vi "Save_Ensight_Case.vi"() -> (5 "Plug in titles":string[](array[string]), 7 "Plug in values":string[](array[string]))   [LabVIEW 2011]
uses:
  Globals/Meas_global.vi
  <vilib>/Analysis/NI_AALBase.lvlib
panel:
  out "Channel Varaibles":string[](array[string])
  out "Variable Names":string[](array[string])
  out "File Paths":path[](array[path])
  out "Results Folder Exists?":bool
  # "You must have just these two indicators on the connector pane of the vi"
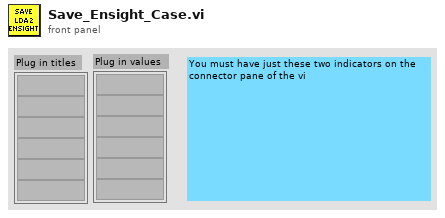
[diagram p1: front panel]
types:
  T1 = typedef "Analysis_info_cluster.ctl" = cluster{"Colour":u32, "Inst type":T2, "Inst name":string, "Symbol":string, "Code name":string, "Extra Info":string, "Inst Array":T3, "Index":i32, "Voltage Index":i32, "Extra Titles":string[], "Extra Values":string[], "Eng Values":dbl[], "Time (ms)":dbl[], "Voltage":dbl[], "U":dbl, "u^2":dbl, "u^3":dbl, "u^4":dbl, "Skew_u":dbl, "Kurt_u":dbl, "Sd Error in Mean":dbl, "% u'/U":dbl, "X":dbl, "Y":dbl, "Z":dbl, "Spectra":T4, "Autocorrelation":T4, "Timescale integral to 25%":dbl, "Sd Error in Variance":dbl, "Calib File":path, "Calib Constants":dbl[], "Histogram":T4, "Output Position":bool, "Full Stats":bool, "Weighting":dbl[]}
  T2 = typedef "Inst_type.ctl" = enum16{"Propeller anemometer", "Raw voltage", "Pressure Transducer", "Pitot-static tube", "Preston tube", "Hot wire", "Cross wire 1", "Cross wire 2", "Generic Linear", "Generic Polynomial", "Generic BackPoly", "Fast FID", "Thermocouple", "Cold wire", "Pulsed Wire", "LDA Vel", "LDA Tran time", "LDA Arr time"}
  T3 = typedef "Instrument_Array.ctl" = enum16{"PWA", "LDA", "Analogue"}
  T4 = typedef "XY_Plot_Cluster.ctl" = cluster{"First Name":string, "Second Name":string, "X axis name":string, "Y axis name":string, "X array":dbl[], "Y array":dbl[]}
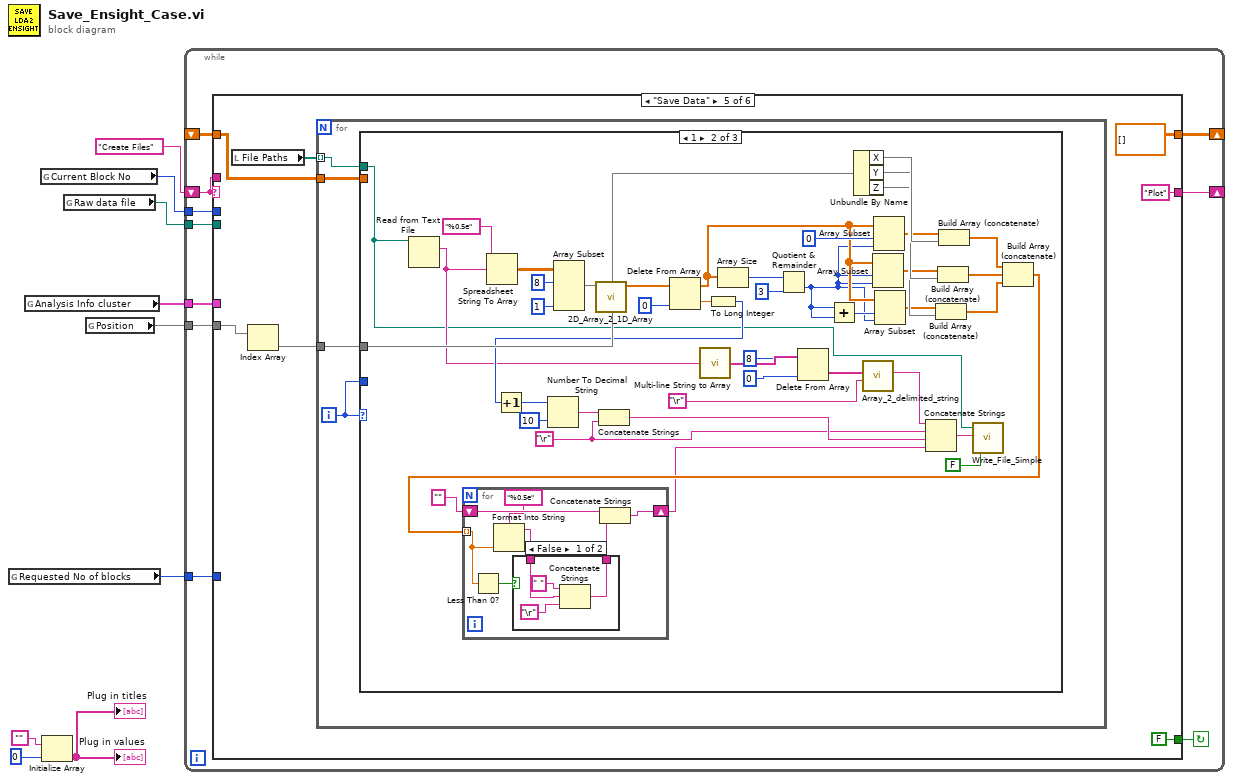
[diagram p0: block diagram]
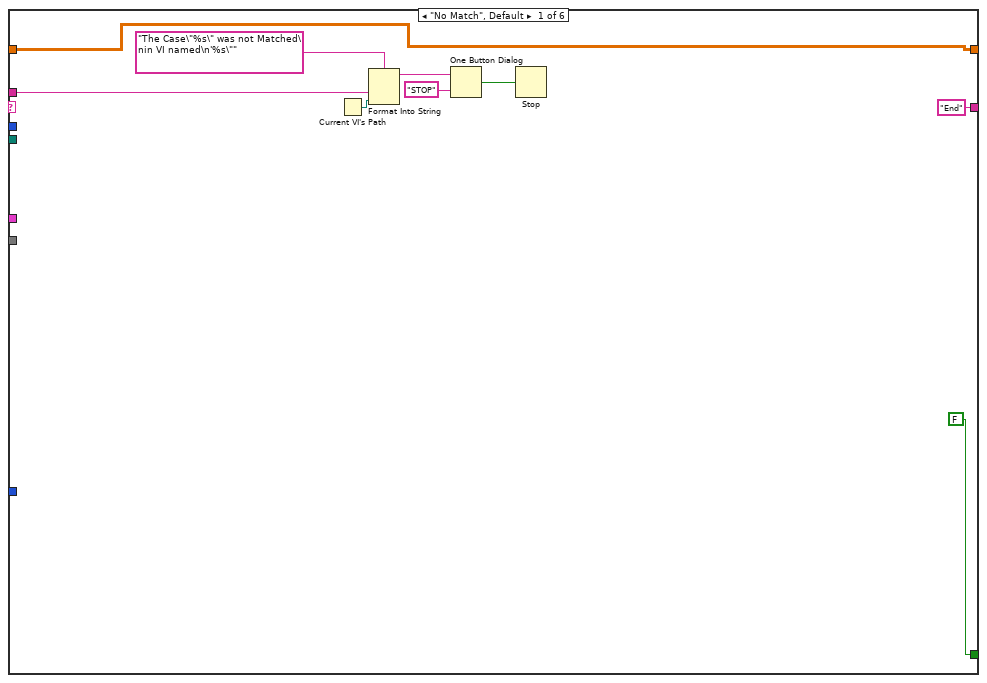
[diagram p2: hidden frame]
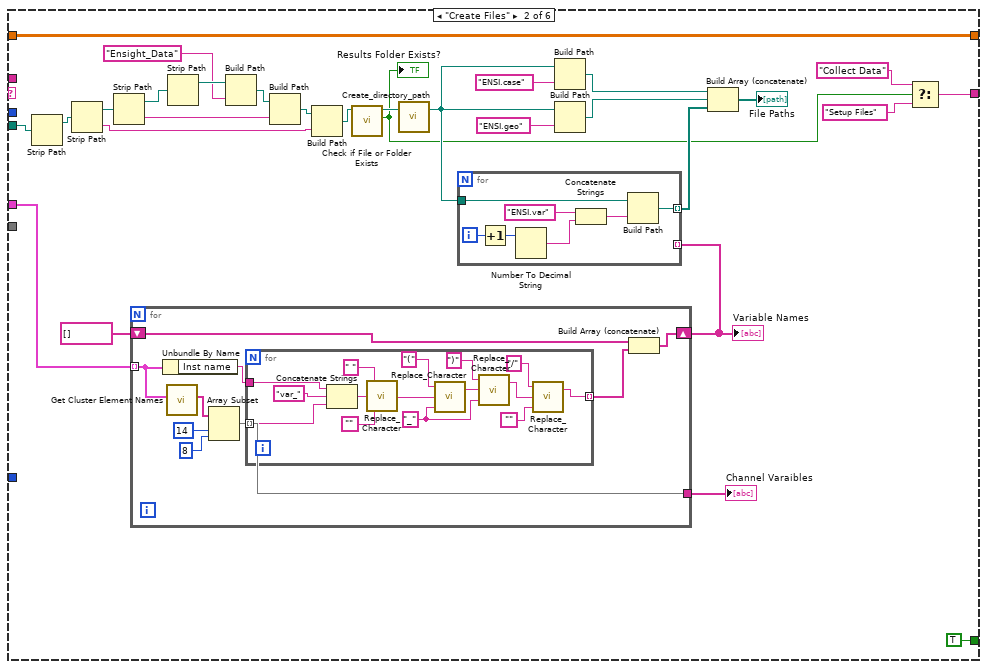
[diagram p3: hidden frame]
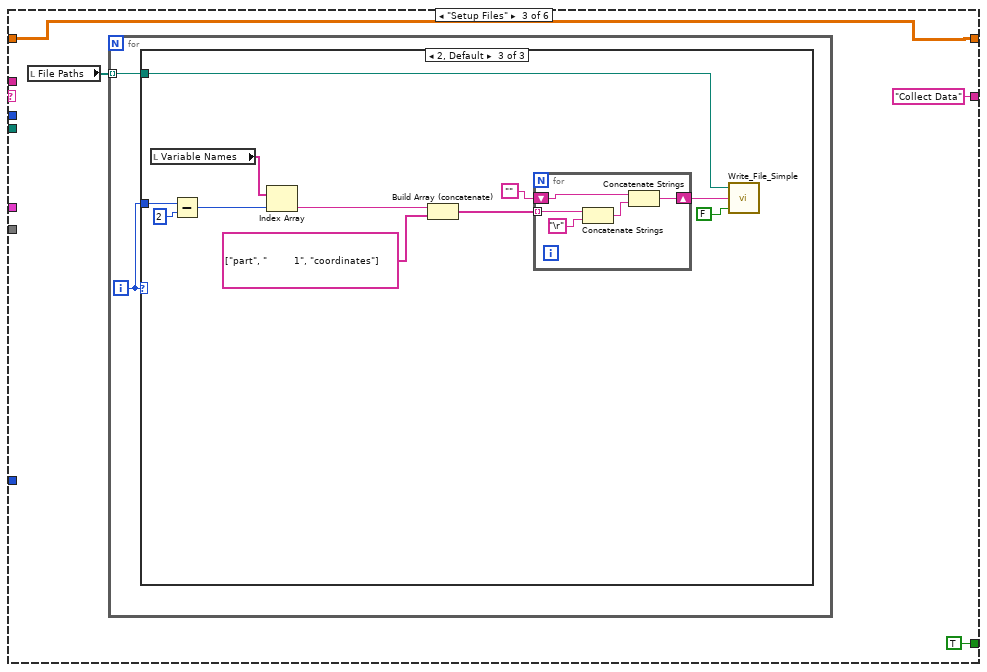
[diagram p4: hidden frame]
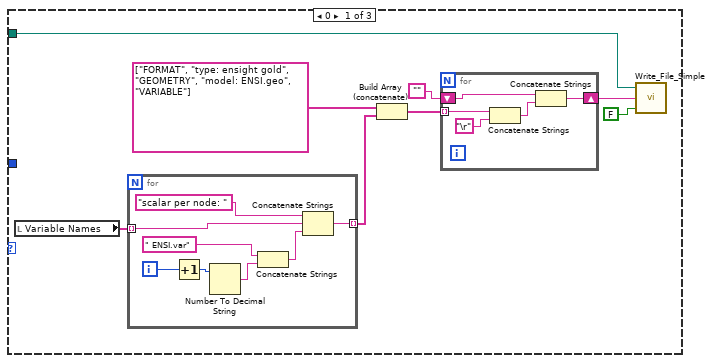
[diagram p5: hidden frame]
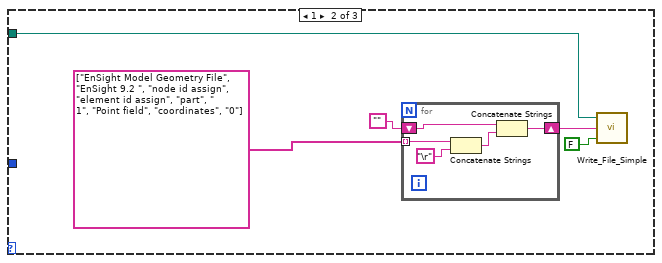
[diagram p6: hidden frame]
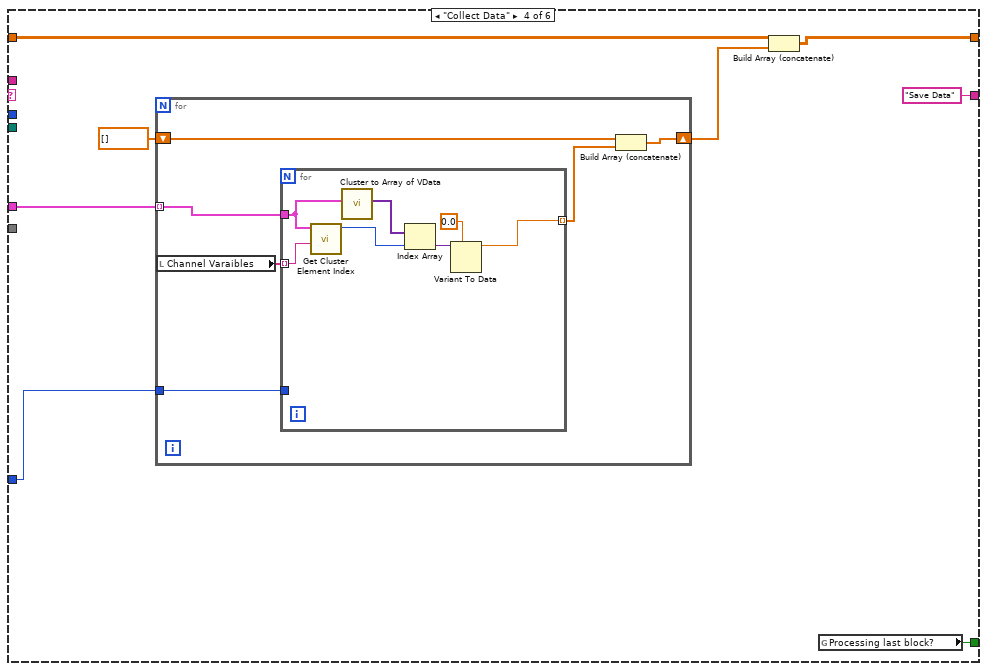
[diagram p7: hidden frame]
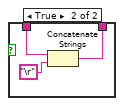
[diagram p9: hidden frame]
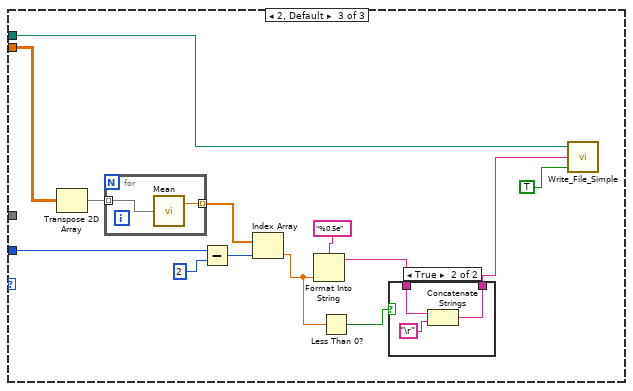
[diagram p10: hidden frame]
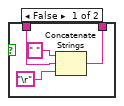
[diagram p11: hidden frame]
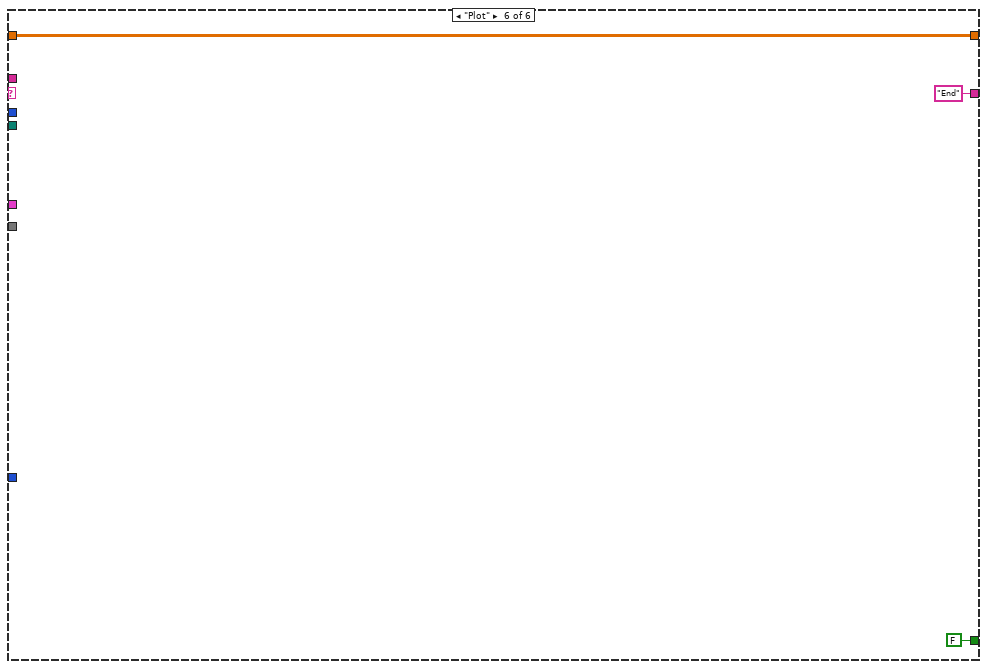
[diagram p12: hidden frame]
diagram:
  n1 = global read "Meas_global.vi" "Requested No of blocks"() -> (w2:i32)
  n2 = global read "Meas_global.vi" "Analysis Info cluster"() -> (w3:T1[])
  n3 = global read "Meas_global.vi" "Current Block No"() -> (w5:i32)
  n4 = Initialize Array("", 0) -> (→"Plug in values" →"Plug in titles":string[])
  n5 = global read "Meas_global.vi" "Raw data file"() -> (w4:path)
  n6 = global read "Meas_global.vi" "Position"() -> (w1)
  n7 = while {
    shift-left: "Create Files" -> [w19]
    shift-right: [w18] -> _
    tunnel: w5 -> [w16]
    tunnel: w4 -> [w15]
    tunnel: w3 -> [w14]
    tunnel: w2 -> [w13]
    tunnel: w1 -> [w12]
    shift-right: [w11] -> _
    shift-left: _ -> [w10]
    stop <- w17 continue-if-true
    n8 = case shown="\"Save Data\"" w19 {
      tunnel: ["End" ("t") w40 "Collect Data" ("t") "Save Data" ("t") "Plot" ("t") "End" ("t")] -> w18
      tunnel: w19 -> [w24 _ _ _ _ _]
      tunnel: [FALSE TRUE ("Processing last block?") TRUE ("Processing last block?") w149 FALSE ("Processing last block?") FALSE ("Processing last block?")] -> w17
      tunnel: w16 -> [_ _ _ _ _ _]
      tunnel: w15 -> [_ w57 _ _ _ _]
      tunnel: w14 -> [_ w36 _ w148 _ _]
      tunnel: w13 -> [_ _ _ w147 _ _]
      tunnel: w12 -> [_ _ _ _ w166 _]
      tunnel: [w20 w29 w89 w143 dbl[][] [] w253] -> w11
      tunnel: w10 -> [w20 w29 w89 w142 w163 w253]
      frame "No Match", Default {
        n9 = Current VI's Path() -> (path=w23:path)
        n10 = Format Into String(format string="The Case\"%s\" was not Matched\nin VI named\n'%s\"" ("Format String"), w24, w23) -> (resulting string=w27:string)  [unwired: 2 in, 1 out]
        n11 = One Button Dialog(message=w27, button name ("OK")="STOP") -> (true=w25:bool)
        n12 = Stop(stop? (T)=w25) -> ()
      }
      frame "Create Files" {
        n13 = Strip Path(path=w57) -> (stripped path=w56:path)  [unwired: 1 out]
        n14 = Strip Path(path=w56) -> (stripped path=w55:path, name=w30:string)
        n15 = Strip Path(path=w55) -> (stripped path=w54:path, name=w50:string)
        n16 = for {
          tunnel: w36 -> [w58] mode=indexing
          shift-right: [w62] -> w33
          shift-left: string[] [] -> [w60]
          tunnel: [w59] -> w34
          n17 = Unbundle By Name(w58) -> ("Inst name"=w63:string)
          n18 = call "Get Cluster Element Names.vi"("Cluster"=w58) -> ("Element Names"=w66:string[])  [unwired: 9 in, 1 out]
          n19 = Array Subset(array=w66, index=14, length=8) -> (w59:string[])
          n20 = for {
            tunnel: w59 -> [w81] mode=indexing
            tunnel: w63 -> [w80]
            tunnel: [w68] -> w61 mode=indexing
            w72 = "_" ("Replace with")
            n21 = Concatenate Strings(w80, "var_" ("string"), w81) -> (w78:string)
            n22 = call "Replace_Character.vi"("Replace with"="", "Input String"=w78, "Search For"=" ") -> ("Output string"=w67:string)  [unwired: 1 out]
            n23 = call "Replace_Character.vi"("Replace with"=w72, "Input String"=w67, "Search For"="(") -> ("Output string"=w74:string)  [unwired: 1 out]
            n24 = call "Replace_Character.vi"("Replace with"=w72, "Input String"=w74, "Search For"=")") -> ("Output string"=w71:string)  [unwired: 1 out]
            n25 = call "Replace_Character.vi"("Replace with"="", "Input String"=w71, "Search For"="/") -> ("Output string"=w68:string)  [unwired: 1 out]
          }
          n26 = Build Array (concatenate)(w60, w61) -> (w62:string[])
        }
        "Variable Names" <- w33
        "Channel Varaibles" <- w34
        n27 = Strip Path(path=w54) -> (stripped path=w53:path)  [unwired: 1 out]
        n28 = Build Path(base path=w53, name or relative path="Ensight_Data") -> (appended path=w51:path)
        n29 = Build Path(base path=w51, name or relative path=w50) -> (appended path=w31:path)
        n30 = Build Path(base path=w31, name or relative path=w30) -> (appended path=w32:path)
        n31 = call <vilib>:"Check if File or Folder Exists.vi"("path"=w32) -> ("file or folder exists?"=w39:bool, "dup path"=w49:path)  [unwired: 8 in, 1 out]
        "Results Folder Exists?" <- w39
        n32 = call "Create_directory_path.vi"("Path name"=w49) -> ("Path name Out"=w45:path)  [unwired: 1 in, 1 out]
        n33 = for {
          tunnel: w45 -> [w88]
          tunnel: [w82] -> w42 mode=indexing
          tunnel: w33 -> [_] mode=indexing
          i -> [w87]
          n34 = Increment(x=w87) -> (x+1=w86:i32)
          n35 = Number To Decimal String(number=w86) -> (decimal integer string=w84:string)  [unwired: 1 in]
          n36 = Concatenate Strings("ENSI.var" ("name or relative path"), w84) -> (w83:string)
          n37 = Build Path(base path=w88, name or relative path=w83) -> (appended path=w82:path)
        }
        n38 = Build Path(base path=w45, name or relative path="ENSI.case") -> (appended path=w44:path)
        n39 = Build Path(base path=w45, name or relative path="ENSI.geo") -> (appended path=w43:path)
        n40 = Build Array (concatenate)(w44, w43, w42) -> (→"File Paths":path[])
        n41 = Select(t="Collect Data", s=w39, f="Setup Files" ("t")) -> (s? t:f=w40:string)
      }
      frame "Setup Files" {
        n42 = local read "File Paths"() -> (w91:path[])
        n43 = for {
          tunnel: w91 -> [w94] mode=indexing
          i -> [w93]
          n44 = case shown="2, Default" w93 {
            tunnel: w94 -> [w98 w117 w136]
            tunnel: w93 -> [_ _ w131]
            frame 0 {
              n45 = local read "Variable Names"() -> (w102:string[])
              n46 = for {
                tunnel: w102 -> [w110] mode=indexing
                tunnel: [w108] -> w96 mode=indexing
                i -> [w113]
                n47 = Increment(x=w113) -> (x+1=w114:i32)
                n48 = Number To Decimal String(number=w114) -> (decimal integer string=w111:string)  [unwired: 1 in]
                n49 = Concatenate Strings(" ENSI.var", w111) -> (w109:string)
                n50 = Concatenate Strings("scalar per node: ", w110, w109) -> (w108:string)
              }
              n51 = Build Array (concatenate)(string[] ["FORMAT", "type: ensight gold", "GEOMETRY", "model: ENSI.geo", "VARIABLE"], w96) -> (w95:string[])
              n52 = for {
                tunnel: w95 -> [w107] mode=indexing
                shift-right: [w105] -> w100
                shift-left: "" -> [w103]
                n53 = Concatenate Strings(w107, "\r") -> (w104:string)
                n54 = Concatenate Strings(w103, w104) -> (w105:string)
              }
              n55 = call "Write_File_Simple.vi"("append to file? (new file:F)"=FALSE, "character string"=w100, "file path"=w98) -> ()  [unwired: 2 out]
            }
            frame 1 {
              n56 = for {
                tunnel: string[] ["EnSight Model Geometry File", "EnSight 9.2 ", "node id assign", "element id assign", "part", "         1", "Point field", "coordinates", "0"] -> [w125] mode=indexing
                shift-right: [w123] -> w119
                shift-left: "" -> [w121]
                n57 = Concatenate Strings(w125, "\r") -> (w122:string)
                n58 = Concatenate Strings(w121, w122) -> (w123:string)
              }
              n59 = call "Write_File_Simple.vi"("append to file? (new file:F)"=FALSE, "character string"=w119, "file path"=w117) -> ()  [unwired: 2 out]
            }
            frame 2, Default {
              n60 = local read "Variable Names"() -> (w132:string[])
              n61 = Subtract(x=w131, y=2) -> (x-y=w129:i32)
              n62 = Index Array(array=w132, index=w129) -> (element=w128:string)
              n63 = Build Array (concatenate)(w128, string[] ["part", "         1", "coordinates"]) -> (w126:string[])
              n64 = for {
                tunnel: w126 -> [w141] mode=indexing
                shift-right: [w139] -> w134
                shift-left: "" -> [w137]
                n65 = Concatenate Strings(w141, "\r") -> (w138:string)
                n66 = Concatenate Strings(w137, w138) -> (w139:string)
              }
              n67 = call "Write_File_Simple.vi"("append to file? (new file:F)"=FALSE, "character string"=w134, "file path"=w136) -> ()  [unwired: 2 out]
            }
          }
        }
      }
      frame "Collect Data" {
        n68 = for {
          tunnel: w148 -> [w154] mode=indexing
          tunnel: w147 -> [w155]
          shift-right: [w151] -> w144
          shift-left: dbl[] [] -> [w152]
          n69 = local read "Channel Varaibles"() -> (w153:string[])
          n70 = for {
            tunnel: w155 -> [_]
            tunnel: w154 -> [w160]
            tunnel: w153 -> [w162] mode=indexing
            tunnel: [w156] -> w150 mode=indexing
            n71 = call "Get Cluster Element Index.vi"("Element Name"=w162, "Cluster"=w160) -> ("Element Index"=w161:i32)  [unwired: 9 in]
            n72 = call "Cluster to Array of VData.vi"("Cluster"=w160) -> ("Array of VData"=w159:variant[])  [unwired: 9 in, 1 out]
            n73 = Index Array(array=w159, index=w161) -> (element=w158:variant)
            n74 = Variant To Data(type=0.0, Variant=w158) -> (data=w156:dbl)  [unwired: 1 in, 1 out]
          }
          n75 = Build Array (concatenate)(w152, w150) -> (w151:dbl[])
        }
        n76 = Build Array (concatenate)(w142, w144) -> (w143:dbl[][])
        n77 = global read "Meas_global.vi" "Processing last block?"() -> (w149:bool)
      }
      frame "Save Data" {
        n78 = local read "File Paths"() -> (w167:path[])
        n79 = Index Array(array=w166) -> (element=w165)  [unwired: 1 in]
        n80 = for {
          tunnel: w167 -> [w173] mode=indexing
          tunnel: w165 -> [w172]
          tunnel: w163 -> [w170]
          i -> [w171]
          n81 = case shown="1" w171 {
            tunnel: w173 -> [_ w174 w243]
            tunnel: w172 -> [_ w210 _]
            tunnel: w171 -> [_ _ w242]
            tunnel: w170 -> [_ _ w238]
            frame 0 {
            }
            frame 1 {
              w192 = "\r"
              n82 = Read from Text File(file (use dialog)=w174) -> (text=w207:string)  [unwired: 3 in, 3 out]
              n83 = Spreadsheet String To Array(format string="%0.5e", spreadsheet string=w207) -> (array=w211:dbl[][])  [unwired: 2 in]
              n84 = Array Subset(array=w211, index (row)=8 ("index"), length (col)=1 ("length")) -> (w214:dbl[][])  [unwired: 2 in]
              n85 = call "2D_Array_2_1D_Array.vi"("Array in"=w214) -> ("Array out"=w215:dbl[])  [unwired: 10 in]
              n86 = Delete From Array(array=w215, index=0) -> (deleted portion=w188:dbl, array with subset deleted=w180:dbl[])  [unwired: 1 in]
              n87 = call "Multi-line String to Array.vi"("Multi lined string"=w207) -> ("Array of string lines"=w206:string[])
              n88 = To Long Integer(number=w188) -> (32bit integer=w209:i32)
              n89 = Increment(x=w209) -> (x+1=w203:i32)
              n90 = Number To Decimal String(number=w203, width (-)=i16 10) -> (decimal integer string=w202:string)
              n91 = Concatenate Strings(w202, w192) -> (w193:string)
              n92 = Array Size(array=w180) -> (size(s)=w183:i32)
              n93 = Quotient & Remainder(x=w183, y=3) -> (floor(x/y)=w178:i32)  [unwired: 1 out]
              n94 = Delete From Array(array=w206, length=8 ("index"), index=0) -> (deleted portion=w190:string[])  [unwired: 1 out]
              n95 = Add(x=w178, y=w178) -> (x+y=w179:i32)
              n96 = Unbundle By Name(w210) -> ("X"=w199, "Y"=w198, "Z"=w197)
              n97 = call "Array_2_delimited_string.vi"("delimiter (Tab)"="\r", "Array of Strings"=w190) -> ("delimited string"=w189:string)  [unwired: 9 in]
              n98 = Array Subset(array=w180, index=w178, length=w178) -> (w176:dbl[])
              n99 = Array Subset(array=w180, index=0, length=w178) -> (w177:dbl[])
              n100 = Array Subset(array=w180, index=w179, length=w178) -> (w175:dbl[])
              n101 = Build Array (concatenate)(w175, w197) -> (w194:dbl[])
              n102 = Build Array (concatenate)(w176, w198) -> (w195:dbl[])
              n103 = Build Array (concatenate)(w177, w199) -> (w196:dbl[])
              n104 = Build Array (concatenate)(w196, w195, w194) -> (w187:dbl[])
              n105 = for {
                tunnel: w187 -> [w218] mode=indexing
                shift-right: [w223] -> w185
                shift-left: "" -> [w222]
                n106 = Less Than 0?(x=w218) -> (x < 0?=w217:bool)
                n107 = Format Into String(format string="%0.5e", w218) -> (resulting string=w219:string)  [unwired: 2 in, 1 out]
                n108 = case shown="False" w217 {
                  tunnel: [w225 w229] -> w221
                  tunnel: w219 -> [w226 w228]
                  frame False {
                    n109 = Concatenate Strings(" " ("string"), w226, "\r") -> (w225:string)
                  }
                  frame True {
                    n110 = Concatenate Strings(w228, "\r") -> (w229:string)
                  }
                }
                n111 = Concatenate Strings(w222, w221) -> (w223:string)
              }
              n112 = Concatenate Strings(w189, w192, w193, w185) -> (w201:string)
              n113 = call "Write_File_Simple.vi"("append to file? (new file:F)"=FALSE, "character string"=w201, "file path"=w174) -> ()  [unwired: 2 out]
            }
            frame 2, Default {
              n114 = Transpose 2D Array(2D array=w238) -> (transposed array=w236:dbl[][])
              n115 = for {
                tunnel: w236 -> [w252] mode=indexing
                tunnel: [w251] -> w237 mode=indexing
                n116 = call <vilib>:"Mean.vi"("X"=w252) -> ("mean"=w251:dbl)  [unwired: 1 out]
              }
              n117 = Subtract(x=w242, y=2) -> (x-y=w240:i32)
              n118 = Index Array(array=w237, index=w240) -> (element=w232:dbl)
              n119 = Format Into String(format string="%0.5e", w232) -> (resulting string=w234:string)  [unwired: 2 in, 1 out]
              n120 = Less Than 0?(x=w232) -> (x < 0?=w231:bool)
              n121 = case shown="True" w231 {
                tunnel: [w245 w249] -> w233
                tunnel: w234 -> [w246 w248]
                frame False {
                  n122 = Concatenate Strings(" " ("string"), w246, "\r") -> (w245:string)
                }
                frame True {
                  n123 = Concatenate Strings(w248, "\r") -> (w249:string)
                }
              }
              n124 = call "Write_File_Simple.vi"("append to file? (new file:F)"=TRUE, "character string"=w233, "file path"=w243) -> ()  [unwired: 2 out]
            }
          }
        }
      }
      frame "Plot" {
      }
    }
  }
